vi "ReferenceScanRate.vi"() -> (3 "Scan Rate Ref":refnum<vi>)   [LabVIEW 2016]
panel:
  in  "error in":errorcluster
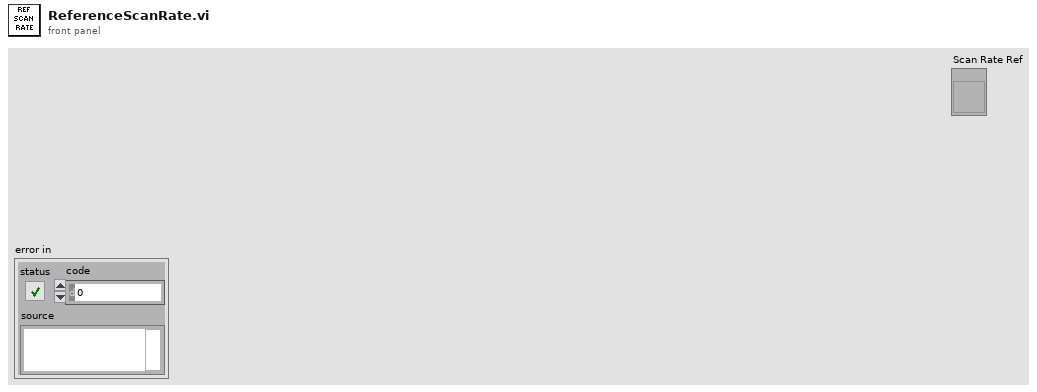
[diagram p1: front panel]
types:
  T1 = enum32{"Bad", "Idle", "Run top level", "Running"}
  T2 = enum32{"Invalid", "Standard", "Closed", "Hidden", "Minimized", "Maximized"}
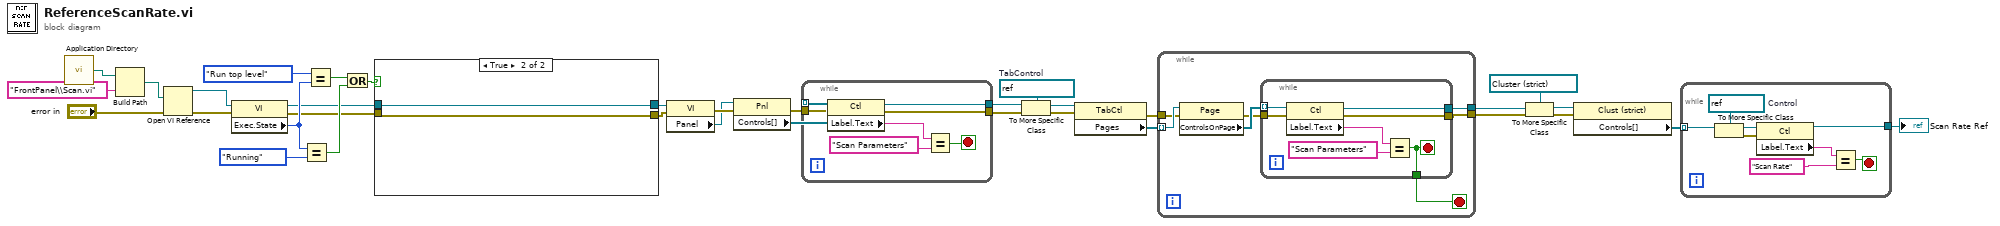
[diagram p0: block diagram]
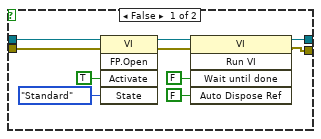
[diagram p2: hidden frame]
diagram:
  w11 = refnum<vi> refnum  # TabControl
  n1 = call <vilib>:"Application Directory.vi"() -> ("Application Directory"=w30:path)
  n2 = Build Path(base path=w30, name or relative path="FrontPanel\\Scan.vi") -> (appended path=w29:path)
  n3 = Open VI Reference(vi path=w29, error in (no error)="error in") -> (vi reference=w20:refnum<vi>, error out=w21:errorcluster)  [unwired: 4 in]
  n4 = property class="VI"(reference=w20, error in=w21) -> (reference out=w19:refnum<vi>, error out=w18:errorcluster, "Exec.State"=w22:T1)
  n5 = Equal?(x=w22, y=T1."Running" ("Execution:State")) -> (x = y?=w23:bool)
  n6 = Equal?(x=T1."Run top level" ("Execution:State"), y=w22) -> (x = y?=w24:bool)
  n7 = Or(x=w24, y=w23) -> (x .or. y?=w17:bool)
  n8 = case shown="True" w17 {
    tunnel: w19 -> [w38 w46]
    tunnel: w18 -> [w37 w45]
    tunnel: [w36 w46] -> w16
    tunnel: [w35 w45] -> w15
    frame False {
      n9 = invoke class="VI" method="FP.Open"(reference=w38, error in=w37, "Activate"=TRUE ("Activate?"), "State"=T2."Standard") -> (reference out=w41:refnum<vi>, error out=w40:errorcluster)  [unwired: 1 in, 3 out]
      n10 = invoke class="VI" method="Run VI"(reference=w41, error in=w40, "Wait until done"=FALSE ("Wait Until Done"), "Auto Dispose Ref"=FALSE ("Auto Dispose Reference")) -> (reference out=w36:refnum<vi>, error out=w35:errorcluster)  [unwired: 1 in, 3 out]
    }
    frame True {
    }
  }
  n11 = property class="VI"(reference=w16, error in=w15) -> (error out=w33:errorcluster, "Panel"=w28:refnum<vi>)  [unwired: 1 out]
  n12 = property class="Pnl"(reference=w28, error in=w33) -> (error out=w34:errorcluster, "Controls[]"=w32:refnum<vi>[])  [unwired: 1 out]
  n13 = while {
    tunnel: w32 -> [w53] mode=indexing
    tunnel: [w51] -> w10
    tunnel: [w50] -> w9
    tunnel: w34 -> [w49]
    stop <- w48 stop-if-true
    n14 = property class="Ctl"(reference=w53, error in=w49) -> (reference out=w51:refnum<vi>, error out=w50:errorcluster, "Label.Text"=w47:string)
    n15 = Equal?(x=w47, y="Scan Parameters") -> (x = y?=w48:bool)
  }
  n16 = To More Specific Class(target class=w11, reference=w10, error in=w9) -> (specific class reference=w8:refnum<vi>, error out=w7:errorcluster)
  n17 = property class="TabCtl"(reference=w8, error in=w7) -> (error out=w5:errorcluster, "Pages"=w6:refnum<vi>[])  [unwired: 1 out]
  n18 = while {
    tunnel: w6 -> [w60] mode=indexing
    tunnel: w5 -> [w57]
    tunnel: [w55] -> w4
    tunnel: [w54] -> w3
    stop <- w56 stop-if-true
    n19 = property class="Page"(reference=w60, error in=w57) -> (error out=w58:errorcluster, "ControlsOnPage"=w59:refnum<vi>[])  [unwired: 1 out]
    n20 = while {
      tunnel: [w66] -> w55
      tunnel: [w65] -> w54
      tunnel: w58 -> [w64]
      tunnel: w59 -> [w63] mode=indexing
      tunnel: [w62] -> w56
      stop <- w62 stop-if-true
      n21 = property class="Ctl"(reference=w63, error in=w64) -> (reference out=w66:refnum<vi>, error out=w65:errorcluster, "Label.Text"=w61:string)
      n22 = Equal?(x=w61, y="Scan Parameters") -> (x = y?=w62:bool)
    }
  }
  n23 = To More Specific Class(target class=refnum<vi> refnum ("Scan Parameters"), reference=w4, error in=w3) -> (specific class reference=w14:refnum<vi>, error out=w13:errorcluster)
  n24 = property class="Clust (strict)"(reference=w14, error in=w13) -> ("Controls[]"=w12:refnum<vi>[])  [unwired: 2 out]
  n25 = while {
    tunnel: w12 -> [w75] mode=indexing
    tunnel: [w68] -> w1
    stop <- w69 stop-if-true
    w72 = refnum<vi> refnum  # Control
    n26 = To More Specific Class(target class=w72, reference=w75) -> (specific class reference=w74:refnum<vi>, error out=w73:errorcluster)  [unwired: 1 in]
    n27 = property class="Ctl"(reference=w74, error in=w73) -> (reference out=w68:refnum<vi>, "Label.Text"=w71:string)  [unwired: 1 out]
    n28 = Equal?(x=w71, y="Scan Rate") -> (x = y?=w69:bool)
  }
  "Scan Rate Ref" <- w1
